vi "Show Animated Busy Icon with Message.vi"(4 "Animated Busy Icon Control Name (Animated Busy Icon)":string="Animated Busy Icon", 5 "Already active? (F)":bool, 6 "Message Control Name (Message)":string="Message", 7 "Message":string, 9 "Error In":errorcluster, 11 "Target VI Refnum":refnum<vi>) -> (1 "Error Out":errorcluster)   [LabVIEW 2021, in "GUI.lvlib"]
doc: "This VI uses error in normally (doesn't do anything if there is an error in) and passes through the error in (ignores additional internal errors)."
uses:
  GUI/GUI.lvlib
  Error/Error.lvlib
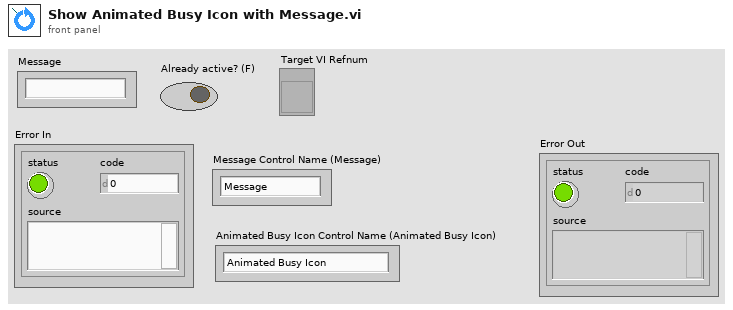
[diagram p1: front panel]
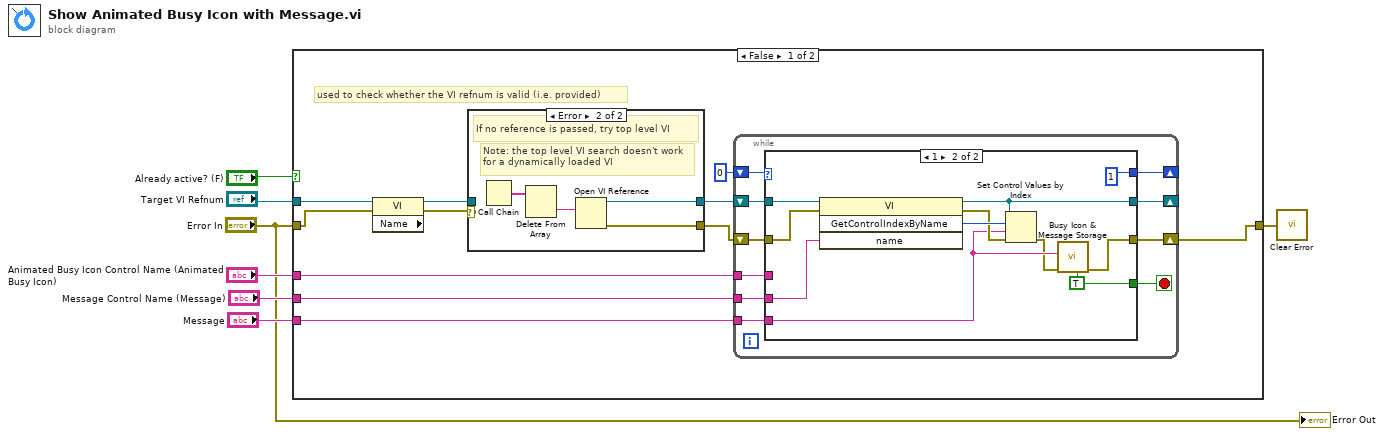
[diagram p0: block diagram]
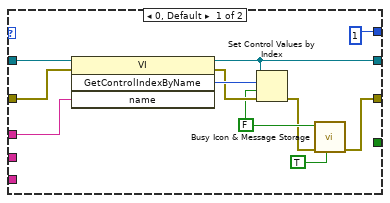
[diagram p3: hidden frame]
diagram:
  n1 = case shown="False" "Already active? (F)" {
    tunnel: [w16 w57] -> w1
    tunnel: "Message Control Name (Message)" -> [w14 _]
    tunnel: "Animated Busy Icon Control Name (Animated Busy Icon)" -> [w13 _]
    tunnel: "Message" -> [w12 _]
    tunnel: "Target VI Refnum" -> [w11 _]
    tunnel: "Error In" -> [w8 w57]
    frame False {
      # "used to check whether the VI refnum is valid (i.e. provided)"
      n2 = property class="VI" props=["Name"](reference=w11, error in=w8) -> (reference out=w9:refnum<vi>, error out=w10:errorcluster)  [unwired: 1 out]
      n3 = case shown="Error" w10 {
        selector: w10 -> [w19 _]
        tunnel: [w19 w24] -> w18
        tunnel: [w20 w23] -> w17
        tunnel: w9 -> [w20 _]
        frame No Error {
        }
        frame Error {
          # "Note: the top level VI search doesn't work for a dynamically loaded VI"
          # "If no reference is passed, try top level VI"
          n4 = Call Chain() -> (call chain=w21:string[])
          n5 = Delete From Array(array=w21) -> (deleted portion=w22:string)  [unwired: 2 in, 1 out]
          n6 = Open VI Reference(vi path=w22) -> (vi reference=w23:refnum<vi>, error out=w24:errorcluster)  [unwired: 5 in]
        }
      }
      n7 = while {
        shift-right: [w31] -> w16
        shift-left: w18 -> [w34]
        shift-right: [w32] -> _
        shift-left: w17 -> [w33]
        shift-right: [w29] -> _
        shift-left: 0 -> [w30]
        tunnel: w14 -> [w27]
        tunnel: w13 -> [w26]
        tunnel: w12 -> [w25]
        stop <- w28 stop-if-true
        n8 = case shown="1" w30 {
          tunnel: w34 -> [w43 w54]
          tunnel: w33 -> [w42 w53]
          tunnel: [w41 w52] -> w32
          tunnel: [w36 w47] -> w31
          tunnel: [1 1] -> w29
          tunnel: [_ w46] -> w28
          tunnel: w27 -> [_ w50]
          tunnel: w26 -> [w39 _]
          tunnel: w25 -> [_ w49]
          frame 0, Default {
            w38 = FALSE ("Visible")
            n9 = invoke class="VI" method="GetControlIndexByName"(reference=w42, error in=w43, "name"=w39) -> (reference out=w41:refnum<vi>, error out=w44:errorcluster, "GetControlIndexByName"=w45:i32)  [unwired: 1 in, 1 out]
            n10 = Set Control Values by Index(0:w41, 1:w45, 2:w38, 3:w44) -> (11:w37:errorcluster)
            n11 = call "Busy Icon & Message Storage.vi"("Get(F)/Set Busy Icon"=TRUE, "Error In"=w37, "Busy Icon Status (F = busy)"=w38) -> ("Error Out"=w36:errorcluster)  [unwired: 6 in, 2 out]
          }
          frame 1 {
            w46 = TRUE ("Get(F)/Set Message")
            n12 = invoke class="VI" method="GetControlIndexByName"(reference=w53, error in=w54, "name"=w50) -> (reference out=w52:refnum<vi>, error out=w55:errorcluster, "GetControlIndexByName"=w56:i32)  [unwired: 1 in, 1 out]
            n13 = Set Control Values by Index(0:w52, 1:w56, 2:w49, 3:w55) -> (11:w48:errorcluster)
            n14 = call "Busy Icon & Message Storage.vi"("Get(F)/Set Message"=w46, "Error In"=w48, "Message String"=w49) -> ("Error Out"=w47:errorcluster)  [unwired: 6 in, 2 out]
          }
        }
      }
    }
    frame True {
    }
  }
  n15 = call "Clear Error.vi"("Error In"=w1) -> ()  [unwired: 8 in, 1 out]
  "Error Out" <- "Error In"
